vi "GetStateData.vi"(8 "error in (no error)":errorcluster, 11 "Exit in":refnum<class "Exit.lvclass">) -> (0 "error out":errorcluster, 1 "Data":string, 2 "State":string, 3 "Exit out":refnum<class "Exit.lvclass">)   [LabVIEW 2020, in "UpstreamMsg.lvlib" / "Exit.lvclass"]
uses:
  Exit.lvclass
  Exit.lvclass/Exit.ctl
  f67ddd79-9209-413a-b458-704e15650e02.vi
  <vilib>/JDP Science/JSONtext/Variant to JSON Text.vi
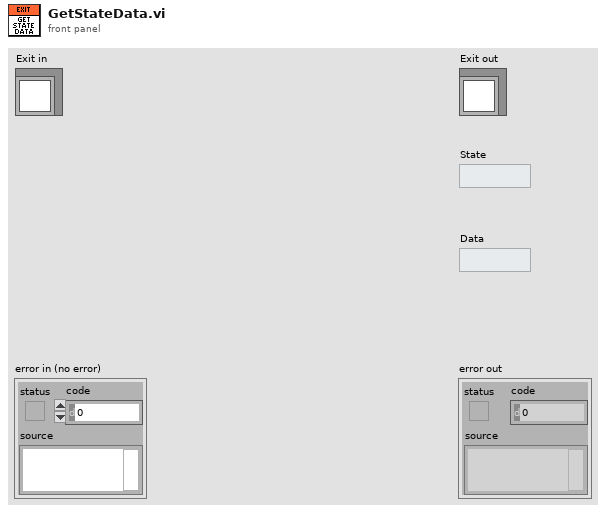
[diagram p1: front panel]
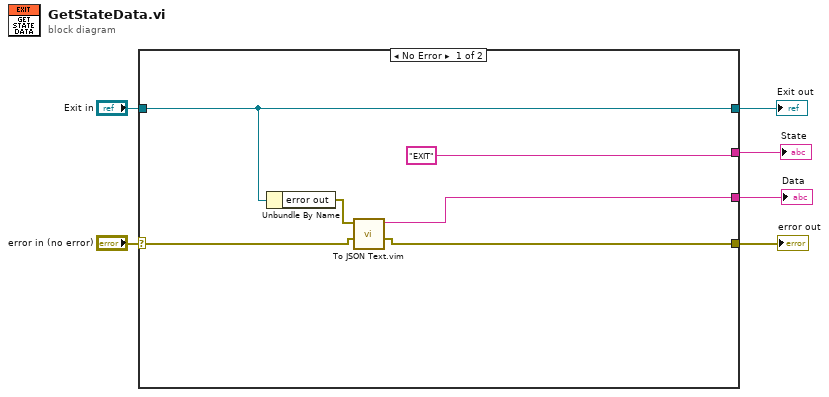
[diagram p0: block diagram]
diagram:
  n1 = case shown="No Error" "error in (no error)" {
    selector: "error in (no error)" -> [w11 w14]
    tunnel: [w10 w14] -> w6
    tunnel: [w8 w13] -> w5
    tunnel: "Exit in" -> [w8 w13]
    tunnel: [w9 _] -> w2
    tunnel: ["EXIT" ("State 2") _] -> w1
    frame No Error {
      n2 = Unbundle By Name(w8) -> ("error out"=w7:errorcluster)
      n3 = call "To JSON Text.vim"("error in (no error)"=w11, "Anything"=w7) -> ("error out"=w10:errorcluster, "<JSON>"=w9:string)  [unwired: 8 in]
    }
    frame Error {
    }
  }
  "error out" <- w6
  "Exit out" <- w5
  "State" <- w1
  "Data" <- w2
